vi "GearLoading.vi"(11 "Activate":bool) -> ()   [LabVIEW 2016]
uses:
  <vilib>/Rock Robotics/WPI/Solenoid/WPI_SolenoidSetEnum.vi
  <vilib>/Rock Robotics/WPI/Solenoid/Deprecated/WPI_SolenoidGetBool.vi
  Robot Global Data.vi
  <vilib>/Rock Robotics/Network Tables/NT Write Boolean.vi
panel:
  in  "Solinoid Stat":bool
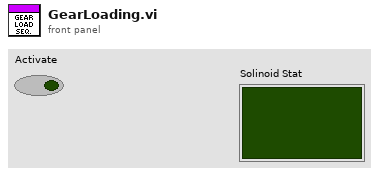
[diagram p1: front panel]
types:
  T1 = typedef "WPI_SwitchDevRef.ctl" = cluster{"DevStatus":errorcluster, "DIO Channel":T2, "CntIndex":T3, "Normally Closed":bool}
  T2 = typedef "FPGA_DIOChannel.ctl" = enum8{"DIO 0", "DIO 1", "DIO 2", "DIO 3", "DIO 4", "DIO 5", "DIO 6", "DIO 7", "DIO 8", "DIO 9", "DIO MXP 0", "DIO MXP 1", "DIO MXP 2", "DIO MXP 3", "DIO MXP 4", "DIO MXP 5", "DIO MXP 6", "DIO MXP 7", "DIO MXP 8", "DIO MXP 9", "DIO MXP 10", "DIO MXP 11", "DIO MXP 12", "DIO MXP 13", "DIO MXP 14", "DIO MXP 15", "SPI Port CS1", "SPI Port CS2", "SPI Port CS3", "SPI Port MISO", "SPI Port MOSI", "Invalid"}
  T3 = typedef "FPGA_CounterCtrSystemIndex.ctl" = enum8{"Ctr 0", "Ctr 1", "Ctr 2", "Ctr 3", "Ctr 4", "Ctr 5", "Ctr 6", "Ctr 7", "Invalid"}
  T4 = typedef "WPI_SolenoidDevRef.ctl" = cluster{"DevStatus":errorcluster, "Pneumatics Control Module":u8, "Forward Solenoid Channel":T5, "Reverse Solenoid Channel":T5}
  T5 = typedef "WPI_SolenoidChannel.ctl" = enum8{"Solenoid 0", "Solenoid 1", "Solenoid 2", "Solenoid 3", "Solenoid 4", "Solenoid 5", "Solenoid 6", "Solenoid 7", "Invalid"}
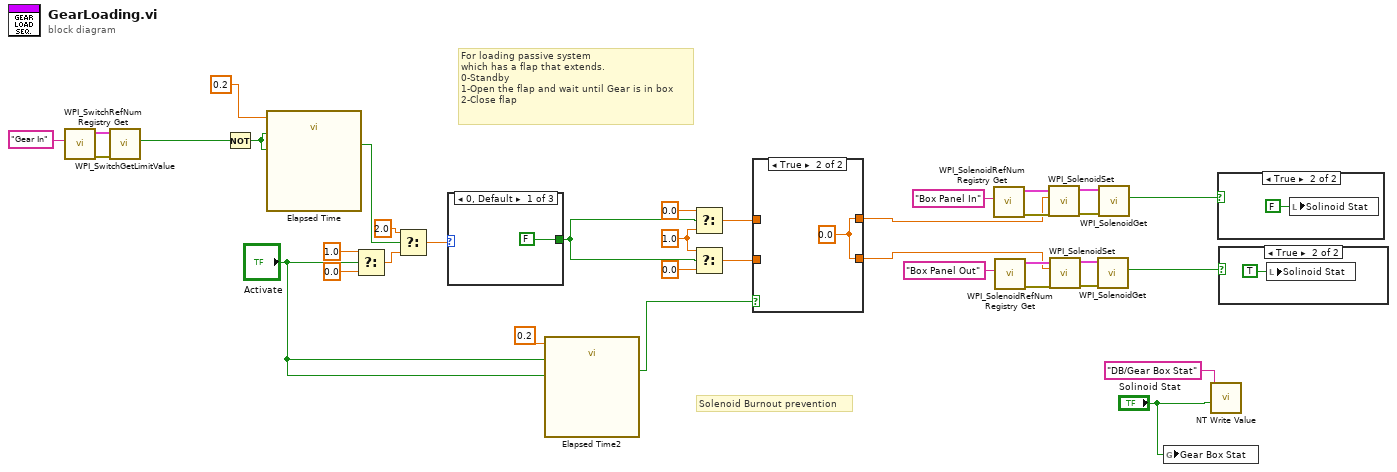
[diagram p0: block diagram]
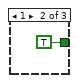
[diagram p5: hidden frame]
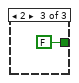
[diagram p6: hidden frame]
diagram:
  w16 = 1.0 ("f")
  # "Solenoid Burnout prevention"
  # "For loading passive system\nwhich has a flap that extends.\n0-Standby\n1-Open the flap and wait until Gear is in box\n2-Close flap"
  n1 = call <vilib>:"WPI_SwitchRefNum Registry Get.vi"("refnum name"="Gear In") -> ("error out"=w30:errorcluster, "SwitchDevRef"=w31:T1)  [unwired: 9 in]
  n2 = call <vilib>:"WPI_SwitchGetLimitValue.vi"("error in (no error)"=w30, "SwitchDevRef"=w31) -> ("Switch Pressed"=w27:bool)  [unwired: 7 in, 2 out]
  n3 = Not(x=w27) -> (.not. x?=w28:bool)
  n4 = call "Elapsed Time"("Time Target (s)"=0.2, "Reset"=w28, "Auto Reset"=w28) -> ("Time has Elapsed"=w25:bool)  [unwired: 9 in, 7 out]
  n5 = Select(t=1.0, s="Activate", f=0.0) -> (s? t:f=w26:dbl)
  n6 = Select(t=2.0, s=w25, f=w26) -> (s? t:f=w24:dbl)
  n7 = case shown="0, Default" w24 {
    tunnel: [FALSE TRUE FALSE] -> w15
    frame 0, Default {
    }
    frame 1 {
    }
    frame 2 {
    }
  }
  n8 = call "Elapsed Time2"("Time Target (s)"=0.2, "Reset"="Activate", "Auto Reset"="Activate") -> ("Time has Elapsed"=w10:bool)  [unwired: 9 in, 7 out]
  n9 = Select(t=0.0, s=w15, f=w16) -> (s? t:f=w14:dbl)
  n10 = Select(t=w16, s=w15, f=0.0) -> (s? t:f=w13:dbl)
  n11 = case shown="True" w10 {
    tunnel: [w41 w43] -> w19
    tunnel: [w42 w43] -> w20
    tunnel: w14 -> [w42 _]
    tunnel: w13 -> [w41 _]
    frame False {
    }
    frame True {
      w43 = 0.0 ("f")
    }
  }
  n12 = call <vilib>:"WPI_SolenoidRefNum Registry Get.vi"("refnum name"="Box Panel In") -> ("error out"=w37:errorcluster, "SolenoidDevRef"=w36:T4)  [unwired: 9 in]
  n13 = call <vilib>:"WPI_SolenoidRefNum Registry Get.vi"("refnum name"="Box Panel Out") -> ("error out"=w34:errorcluster, "SolenoidDevRef"=w33:T4)  [unwired: 9 in]
  n14 = call-poly <vilib>:"WPI_SolenoidSet.vi"("error in (no error)"=w37, "Value"=w20, "SolenoidDevRef"=w36) -> ("error out"=w8:errorcluster, "SolenoidDevRef"=w7:T4)  [unwired: 7 in]
  n15 = call-poly <vilib>:"WPI_SolenoidSet.vi"("error in (no error)"=w34, "Value"=w19, "SolenoidDevRef"=w33) -> ("error out"=w5:errorcluster, "SolenoidDevRef"=w6:T4)  [unwired: 7 in]
  n16 = call-poly <vilib>:"WPI_SolenoidGet.vi"("error in (no error)"=w5, "SolenoidDevRef"=w6) -> ("Value"=w2:bool)  [unwired: 7 in, 2 out]
  n17 = call-poly <vilib>:"WPI_SolenoidGet.vi"("error in (no error)"=w8, "SolenoidDevRef"=w7) -> ("Value"=w3:bool)  [unwired: 7 in, 2 out]
  n18 = global write "Robot Global Data.vi" "Gear Box Stat"("Solinoid Stat") -> ()
  n19 = call-poly <vilib>:"NT Write Value.vi"("Boolean"="Solinoid Stat", "Name"="DB/Gear Box Stat") -> ()  [unwired: 9 in, 1 out]
  n20 = case shown="True" w3 {
    frame False {
    }
    frame True {
      n21 = local write "Solinoid Stat"(FALSE ("Solinoid Stat")) -> ()
    }
  }
  n22 = case shown="True" w2 {
    frame False {
    }
    frame True {
      n23 = local write "Solinoid Stat"(TRUE ("Solinoid Stat")) -> ()
    }
  }
